vi "Read right in tunnels.vi"(9 "FlatSequenceFrame in":refnum<class "FlatSequenceFrame.lvclass">) -> (3 "FlatSequenceFrame out":refnum<class "FlatSequenceFrame.lvclass">, 4 "right in tunnels":refnum<class "FlatSequenceInnerTunnel.lvclass">[](array[class]))   [LabVIEW 2014, in "FlatSequenceFrame.lvclass"]
uses:
  FlatSequenceFrame.lvclass
  FlatSequenceInnerTunnel/FlatSequenceInnerTunnel.lvclass
  FlatSequenceFrame.lvclass/FlatSequenceFrame.ctl
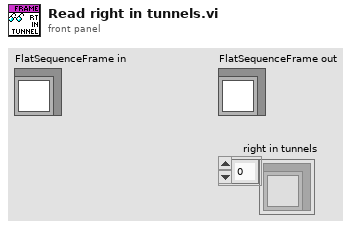
[diagram p1: front panel]
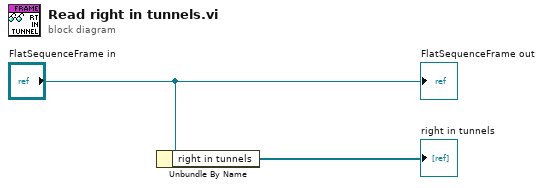
[diagram p0: block diagram]
diagram:
  n1 = Unbundle By Name("FlatSequenceFrame in") -> ("right in tunnels"=→"right in tunnels":refnum<class "FlatSequenceInnerTunnel.lvclass">[])
  "FlatSequenceFrame out" <- "FlatSequenceFrame in"
